vi "ATSpectrograph_getEvent_linearStageInPosition.vi"(8 "error in (no error)":errorcluster, 11 "logevent_linearStageInPosition_Ctl":T1) -> (0 "error out":errorcluster, 2 "function return":i32, 3 "logevent_linearStageInPosition_Ctl out":T1)   [LabVIEW 2016, in "SALLV_ATSpectrograph.lvlib"]
doc: "int ATSpectrograph_shm_getEvent_linearStageInPositionLV(ATSpectrograph_logevent_linearStageInPositionLV *logevent_linearStageInPosition_Ctl );"
uses:
  SALLV_ATSpectrograph.lvlib
  DataTypes/logevent_linearStageInPosition.ctl
  SALLV_ATSpectrograph.so
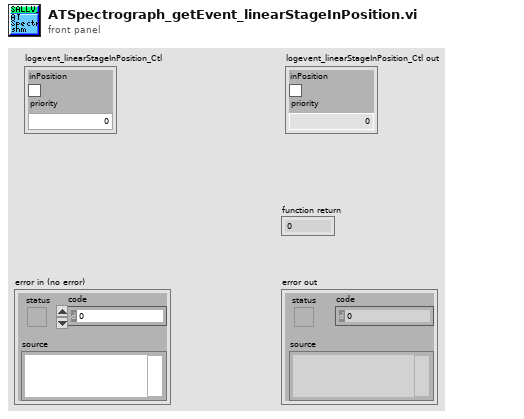
[diagram p1: front panel]
types:
  T1 = typedef "SALLV_ATSpectrograph.lvlib/logevent_linearStageInPosition.ctl" = cluster{"inPosition":bool, "priority":i32}
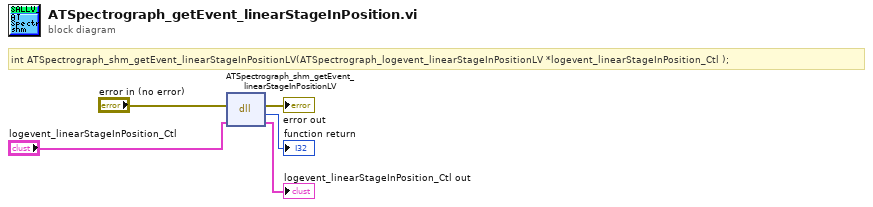
[diagram p0: block diagram]
diagram:
  # "int ATSpectrograph_shm_getEvent_linearStageInPositionLV(ATSpectrograph_logevent_linearStageInPositionLV *logevent_linearStageInPosition_Ctl );"
  n1 = dll-call lib="home/harini/tcs/ts_AtSpectrograph/ts_sallv_AtSpectrograph/SALLV_ATSpectrograph.*" fn="ATSpectrograph_shm_getEvent_linearStageInPositionLV"(error in="error in (no error)", "logevent_linearStageInPosition_Ctl"="logevent_linearStageInPosition_Ctl") -> (error out=→"error out":errorcluster, →"function return":i32, "logevent_linearStageInPosition_Ctl"=→"logevent_linearStageInPosition_Ctl out":T1)  [unwired: 2 in, 1 out]
